vi "Initialize Front Panel.vi"(8 "error in (no error)":errorcluster, 11 "TabbedViewManager in":refnum<class "TabbedViewManager.lvclass">) -> (0 "error out":errorcluster, 3 "TabbedViewManager out":refnum<class "TabbedViewManager.lvclass">)   [LabVIEW 2015, in "TabbedViewManager.lvlib" / "TabbedViewManager.lvclass"]
doc: "<License>\nCopyright © 2017 Composed Systems, LLC | All rights reserved\nwww.composed.io\n\nAuthor: Ethan Stern <ethan.stern@composed.io>\n\nThis software is provided \"AS IS\" WITHOUT WARRANTIES, either express or implied, AND IS FOR EDUCATIONAL PURPOSES ONLY.\n</License>"
uses:
  TabbedViewManager.lvclass
  Framework/IViewManager/IViewManager/IViewManager.lvclass/IViewManager.ctl
  TabbedViewManager.lvclass/TabbedViewManager.ctl
  Framework/IViewable/IViewable Messages/Insert Front Panel Msg/Insert Front Panel Msg.lvclass/Insert Front Panel Msg.ctl
  <vilib>/ActorFramework/Message Enqueuer/Message Enqueuer.lvclass/Message Enqueuer.ctl
  <vilib>/ActorFramework/Message Enqueuer/Enqueue.vi
  <vilib>/ActorFramework/Message Priority Queue/Priority Enqueue.vi
  Framework/IViewManager/IViewManager/IViewManager.lvclass
  Framework/IViewable/IViewable Messages/Insert Front Panel Msg/Insert Front Panel Msg.lvclass
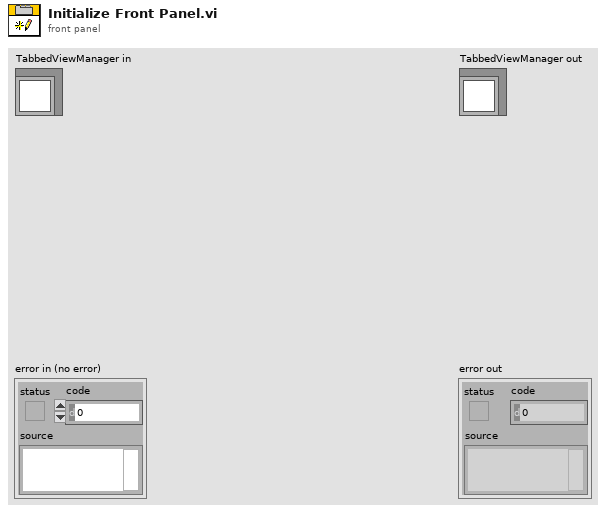
[diagram p1: front panel]
types:
  T1 = enum32{"1", "2", "3", "4", "5", "6", "7", "8", "9", "10"}
  T2 = typedef "IViewable.lvlib/ProtectedSubpanel.lvclass/Protected Subpanel Reference.ctl" = refnum<data-value>
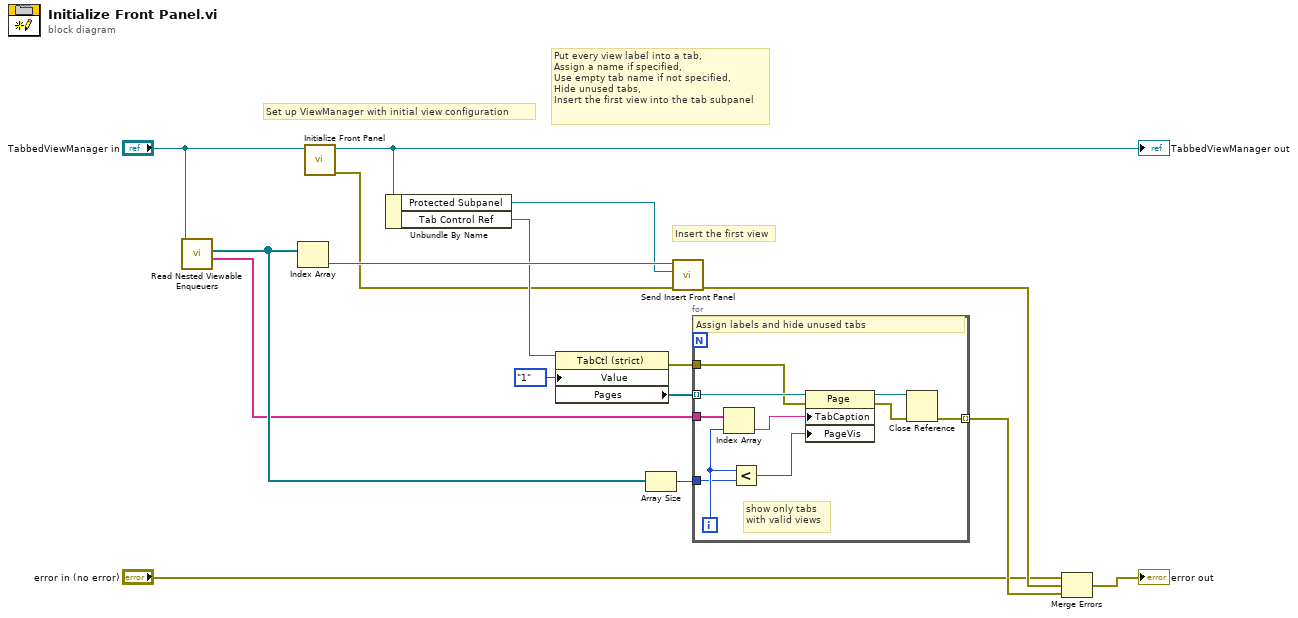
[diagram p0: block diagram]
diagram:
  # "Set up ViewManager with initial view configuration"
  # "Put every view label into a tab,\nAssign a name if specified,\nUse empty tab name if not specified,\nHide unused tabs,\nInsert the first view into the tab subpanel"
  # "Insert the first view"
  n1 = call "Read Nested Viewable Enqueuers.vi"("IViewManager in"="TabbedViewManager in") -> ("Viewable Names"=w1:string[], "Nested Viewable Enqueuers"=w2:refnum<class "Message Enqueuer.lvclass">[])  [unwired: 9 in]
  n2 = Index Array(array=w2) -> (element=w13:refnum<class "Message Enqueuer.lvclass">)  [unwired: 1 in]
  n3 = call-parent "Initialize Front Panel.vi"("IViewable in"="TabbedViewManager in") -> ("error out"=w7:errorcluster, "IViewable out"=w5:refnum<class "TabbedViewManager.lvclass">)  [unwired: 9 in]
  "TabbedViewManager out" <- w5
  n4 = Unbundle By Name(w5) -> ("Protected Subpanel"=w11:T2, "Tab Control Ref"=w12:refnum<vi>)
  n5 = property class="TabCtl (strict)"(reference=w12, "Value"=T1."1") -> (error out=w14:errorcluster, "Pages"=w16:refnum<vi>[])  [unwired: 1 in, 1 out]
  n6 = Array Size(array=w2) -> (size(s)=w15:i32)
  n7 = call "Send Insert Front Panel.vi"("error in (no error)"=w7, "Protected Subpanel"=w11, "Message Enqueuer"=w13) -> ("error out"=w8:errorcluster)  [unwired: 7 in, 1 out]
  n8 = for {
    tunnel: w16 -> [w26] mode=indexing
    tunnel: w1 -> [w25]
    tunnel: w15 -> [w22]
    tunnel: w14 -> [w18]
    tunnel: [w17] -> w9 mode=indexing
    i -> [w23]
    # "show only tabs\nwith valid views"
    # "Assign labels and hide unused tabs"
    n9 = Index Array(array=w25, index=w23) -> (element=w24:string)
    n10 = Less?(x=w23, y=w22) -> (x < y?=w21:bool)
    n11 = property class="Page"(reference=w26, error in=w18, "TabCaption"=w24, "PageVis"=w21) -> (reference out=w20:refnum<vi>, error out=w19:errorcluster)
    n12 = Close Reference(reference=w20, error in (no error)=w19) -> (error out=w17:errorcluster)
  }
  n13 = Merge Errors("error in (no error)", w8, w9) -> (→"error out":errorcluster)
